vi "StateMachine_StageAutomation.vi"() -> ()   [LabVIEW 2021]
uses:
  ProgramData/PI/LabVIEW/Low Level/Communication.llb/Interface Settings.ctl
  C:/Users/csaerome/Documents/PipeJet/PipeJet/Software/bfx_piezo_r13.dll
  Documents/PipeJet/PipeJet/Software/bfx_piezo_r13.dll
panel:
  in  "Automatic2ndRow":bool
  in  "2ndRow":bool
  in  "?":bool
  out "Home Position (mm)":dbl[](array[numeric]) format="%.6f"
  in  "Home":bool
  out "Print Preview":picture
  in  "PrintPreview":bool
  in  "Num. of columns":dbl
  in  "Dist. b/w Columns (mm)":dbl[](array[numeric])
  in  "Num. of wells":dbl
  in  "Dist. b/w wells (mm)":dbl[](array[numeric])
  in  "Dist. b/w cells line (mm)":dbl[](array[numeric])
  in  "Pitch (mm)":dbl[](array[numeric])
  in  "Num. of Drops":dbl
  in  "Z-":bool
  in  "Z+":bool
  in  "Z-Step Size (mm)":dbl[](array[numeric])=[0.0]
  in  "PJ Stroke (%)":dbl
  in  "PJ Str. Velocity":dbl
  in  "SingleHead":bool
  in  "AbsCenter":bool
  in  "Position values (mm)":dbl[](array[numeric]) format="%.6f"
  in  "Y-":bool
  in  "Y+":bool
  in  "X-":bool
  in  "X+":bool
  in  "Y-Step Size (mm)":dbl[](array[numeric])=[0.0]
  out "Error Description":string
  out "error out":errorcluster
  in  "error in (no error)":errorcluster
  in  "X-Step Size (mm)":dbl[](array[numeric])=[0.0]
  out "Conn. \nAxes":string[](array[string])
  in  "Interface settings":T1={"Interface"=0, "Timeout"=5000, "RS232 settings"={"Portnumber"=6, "Baudrate"=5}, "TCP/IP settings"={"Host address/name"="localhost", "Port"=50000, "Board"=0, "TCP/IP Search?"=TRUE}, "USB settings"={"S/N"="", "USB Search?"=TRUE}, "DaisyChain settings"={"Register DC"=FALSE, "DaisyChain Search?"=TRUE, "Device ID"=1}, "DLL for Device"=0} {"DLL for Device" items=["None", "C-843", "C-844", "E-710", "C-843.PM", "C-865", "E-761", "Mercury", "E-755", "E-753", "C-866", "E-712", "E-725", "E-861", "C-867", "E-517", "E-816", "E-709", "PI_GCS2_DLL", "HydraPollux"]; "Interface" items=["RS232", "RS232 DaisyChain", "USB", "USB DaisyChain", "TCP/IP", "TCP/IP DaisyChain", "PCI"]; "RS232 settings"."Portnumber" min=1 step=1; "RS232 settings"."Baudrate" items=["9600", "14400", "19200", "38400", "57600", "115200", "230400", "460800"]}
  # "Initialization"
  # "Setup"
  # "Relative Centering"
  # "Absolute Centering"
  # "Home Settings"
  # "X:"
  # "Y:"
  # "Z:"
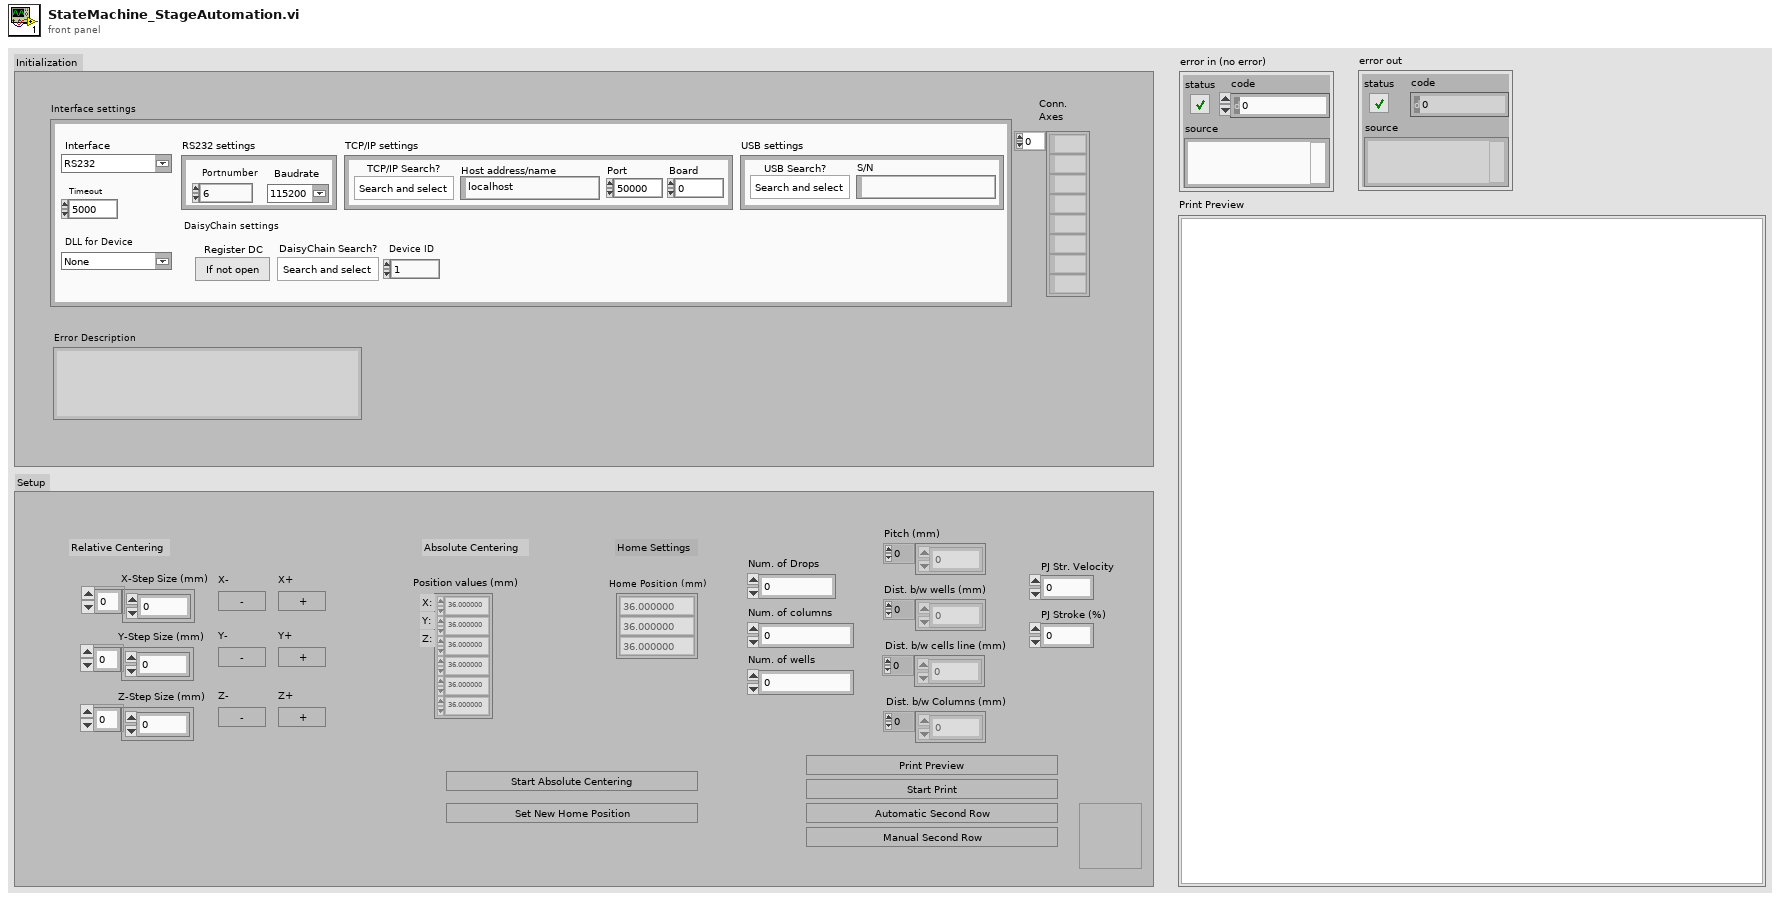
[diagram p1: front panel]
types:
  T1 = typedef "Interface Settings.ctl" = cluster{"Interface":u16, "Timeout":u32, "RS232 settings":cluster{"Portnumber":u8, "Baudrate":u16}, "TCP/IP settings":cluster{"Host address/name":string, "Port":i32, "Board":i32, "TCP/IP Search?":bool}, "USB settings":cluster{"S/N":string, "USB Search?":bool}, "DaisyChain settings":cluster{"Register DC":bool, "DaisyChain Search?":bool, "Device ID":i32}, "DLL for Device":u16}
  T2 = cluster{"Width":u16, "Style":enum32{"Solid", "Dash", "Dot", "DashDot", "DashDotDot"}}
  T3 = enum16{"Do not reference", "Reference switch", "Negative limit switch", "Positive limit switch"}[]
  T4 = cluster{"Dist. b/w cells line (mm)":dbl[], "Pitch (mm)":dbl[], "Num. of Drops":dbl, "Dist. b/w wells (mm)":dbl[], "Num. of wells":dbl, "Num. of columns":dbl, "Dist. b/w Columns (mm)":dbl[]}
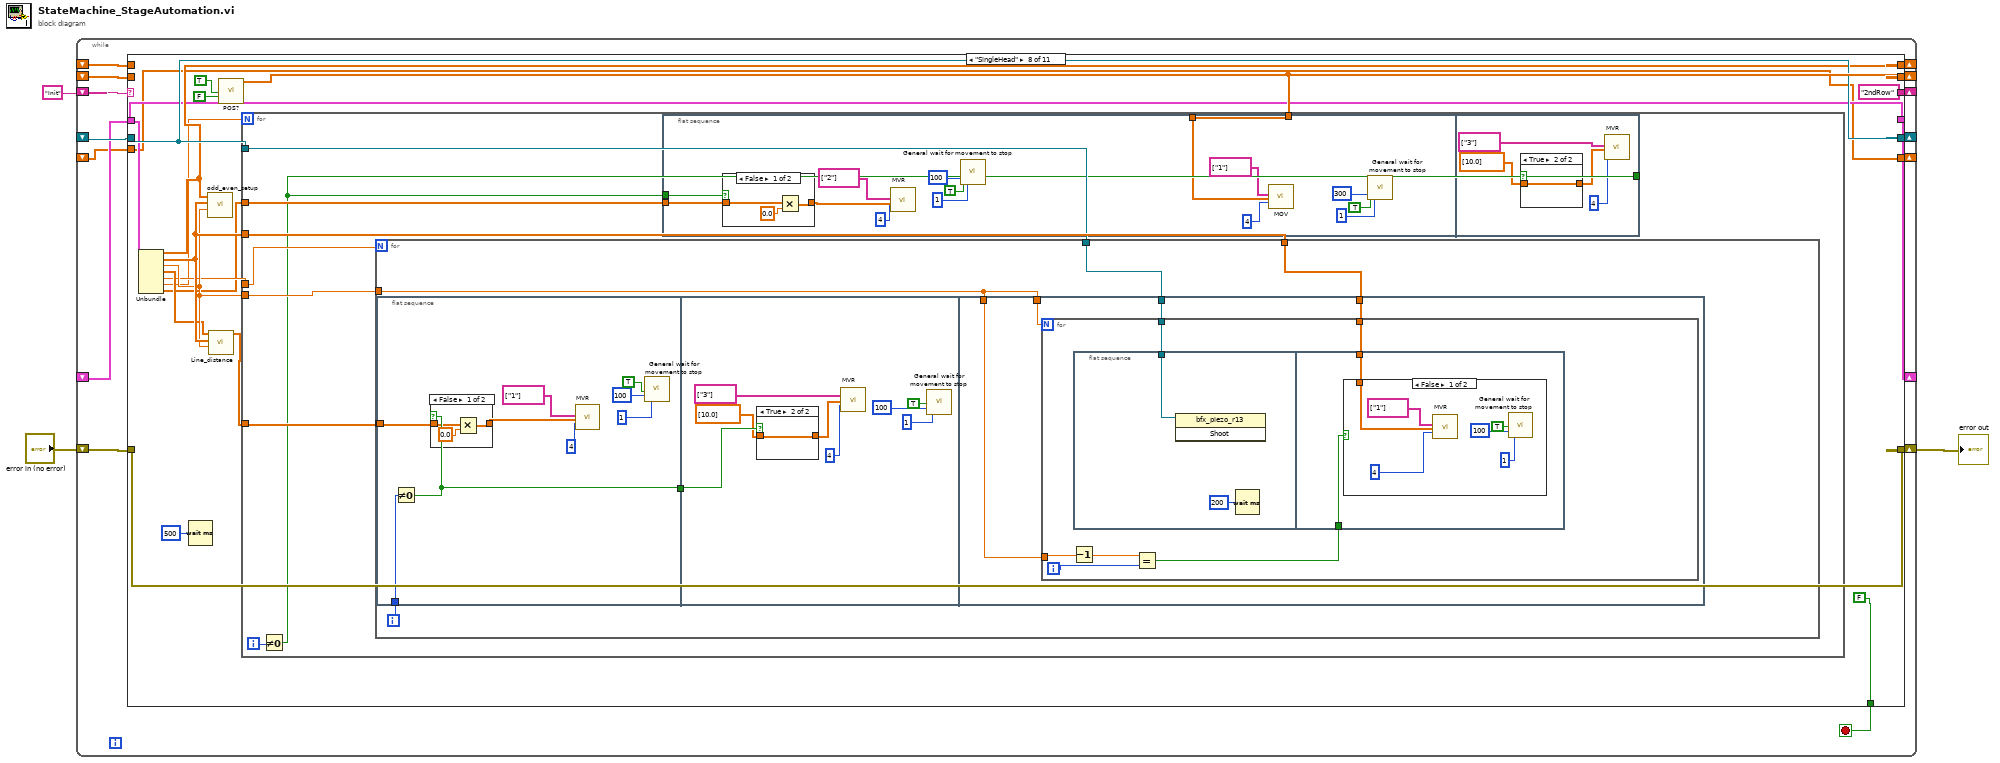
[diagram p0: block diagram]
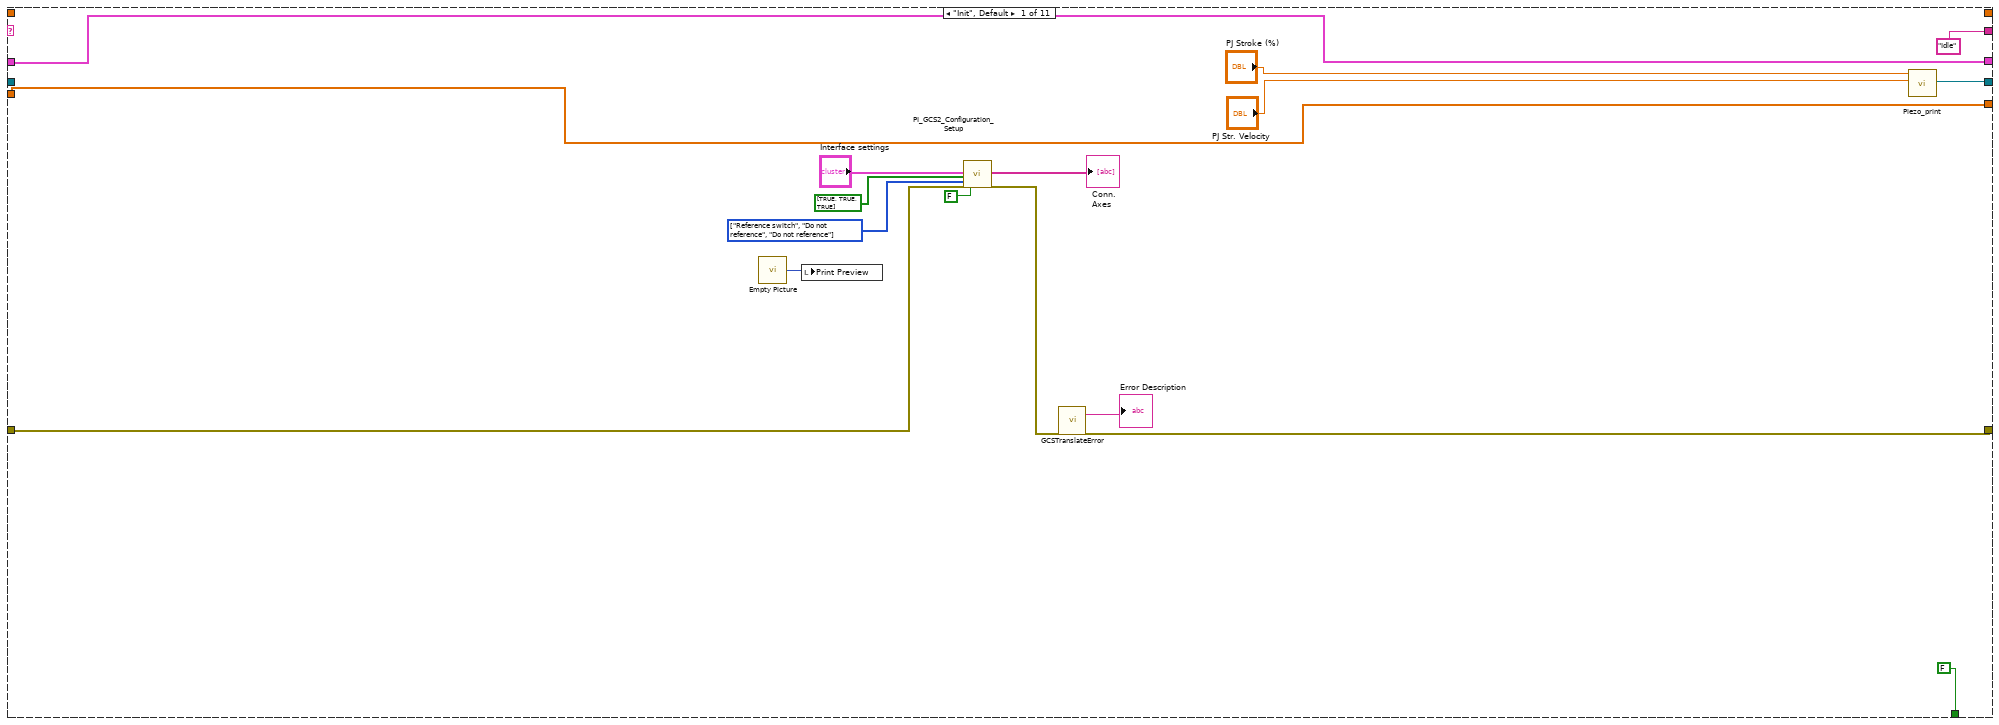
[diagram p2: hidden frame]
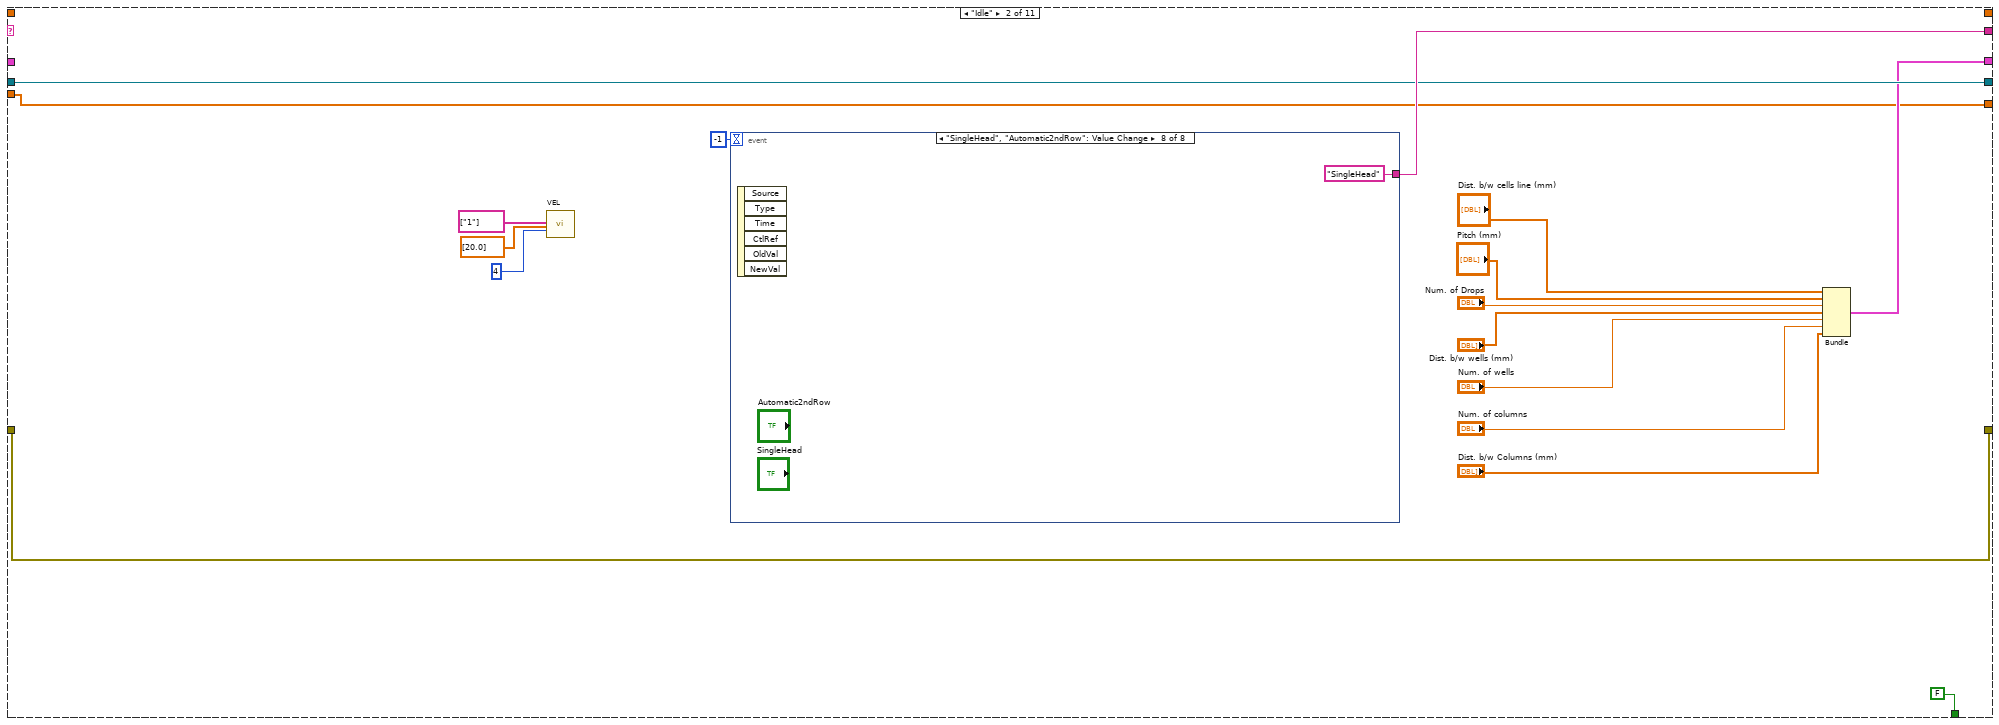
[diagram p3: hidden frame]
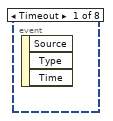
[diagram p4: hidden frame]
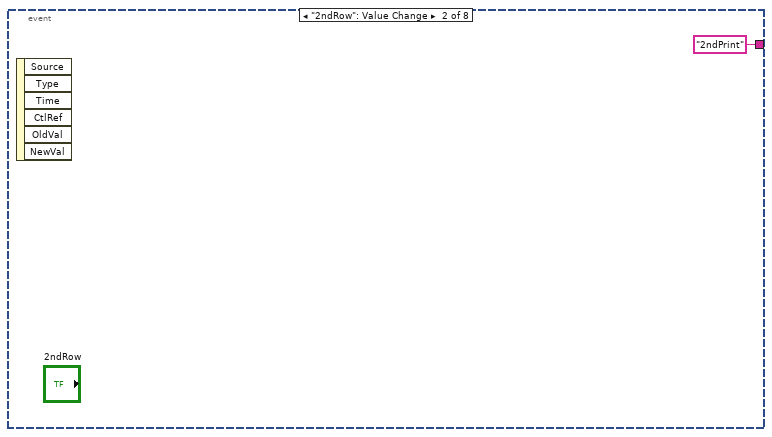
[diagram p5: hidden frame]
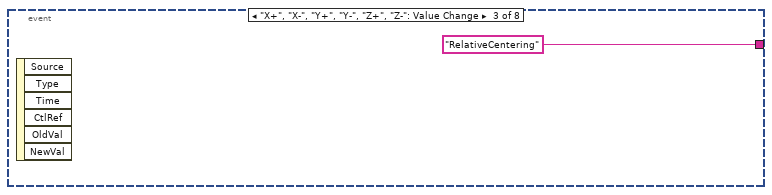
[diagram p6: hidden frame]
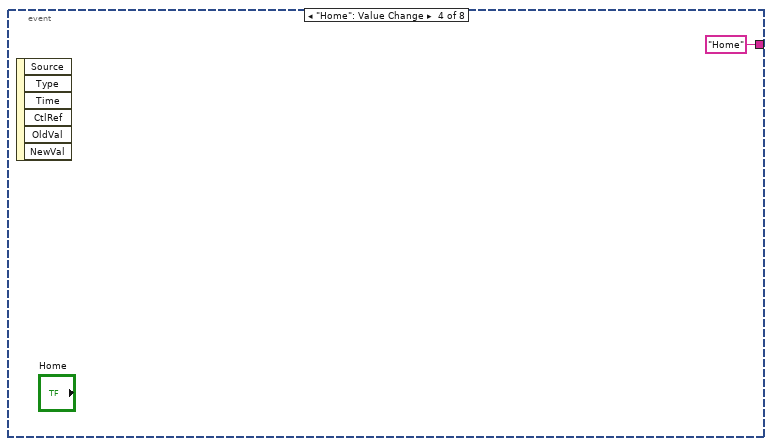
[diagram p7: hidden frame]
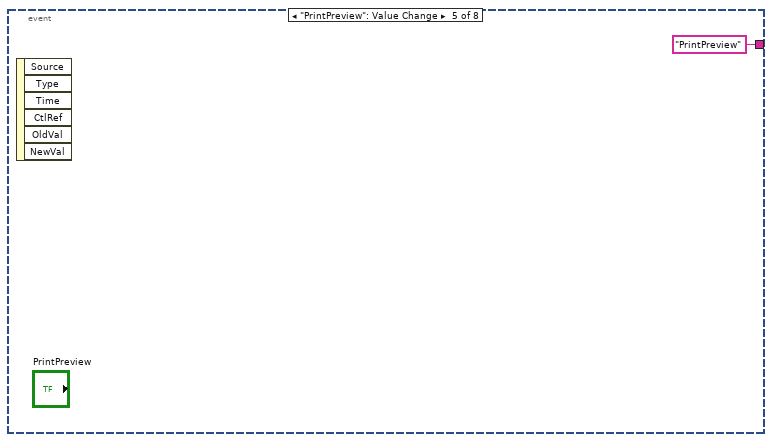
[diagram p8: hidden frame]
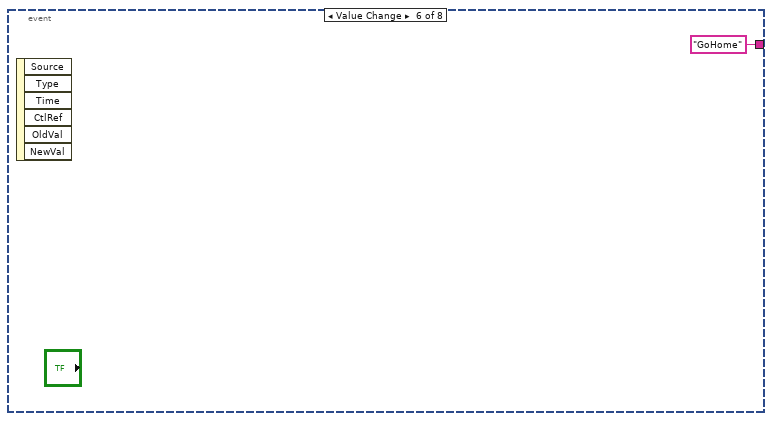
[diagram p9: hidden frame]
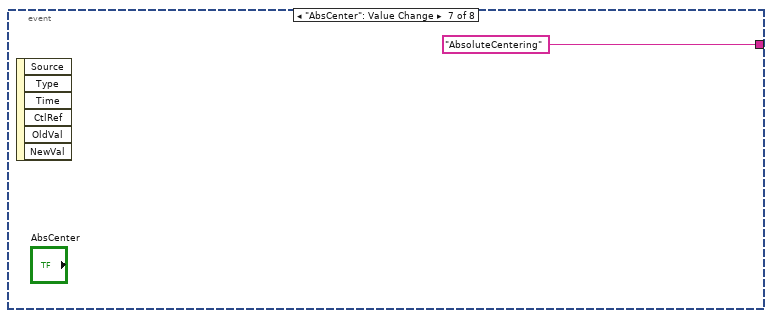
[diagram p10: hidden frame]
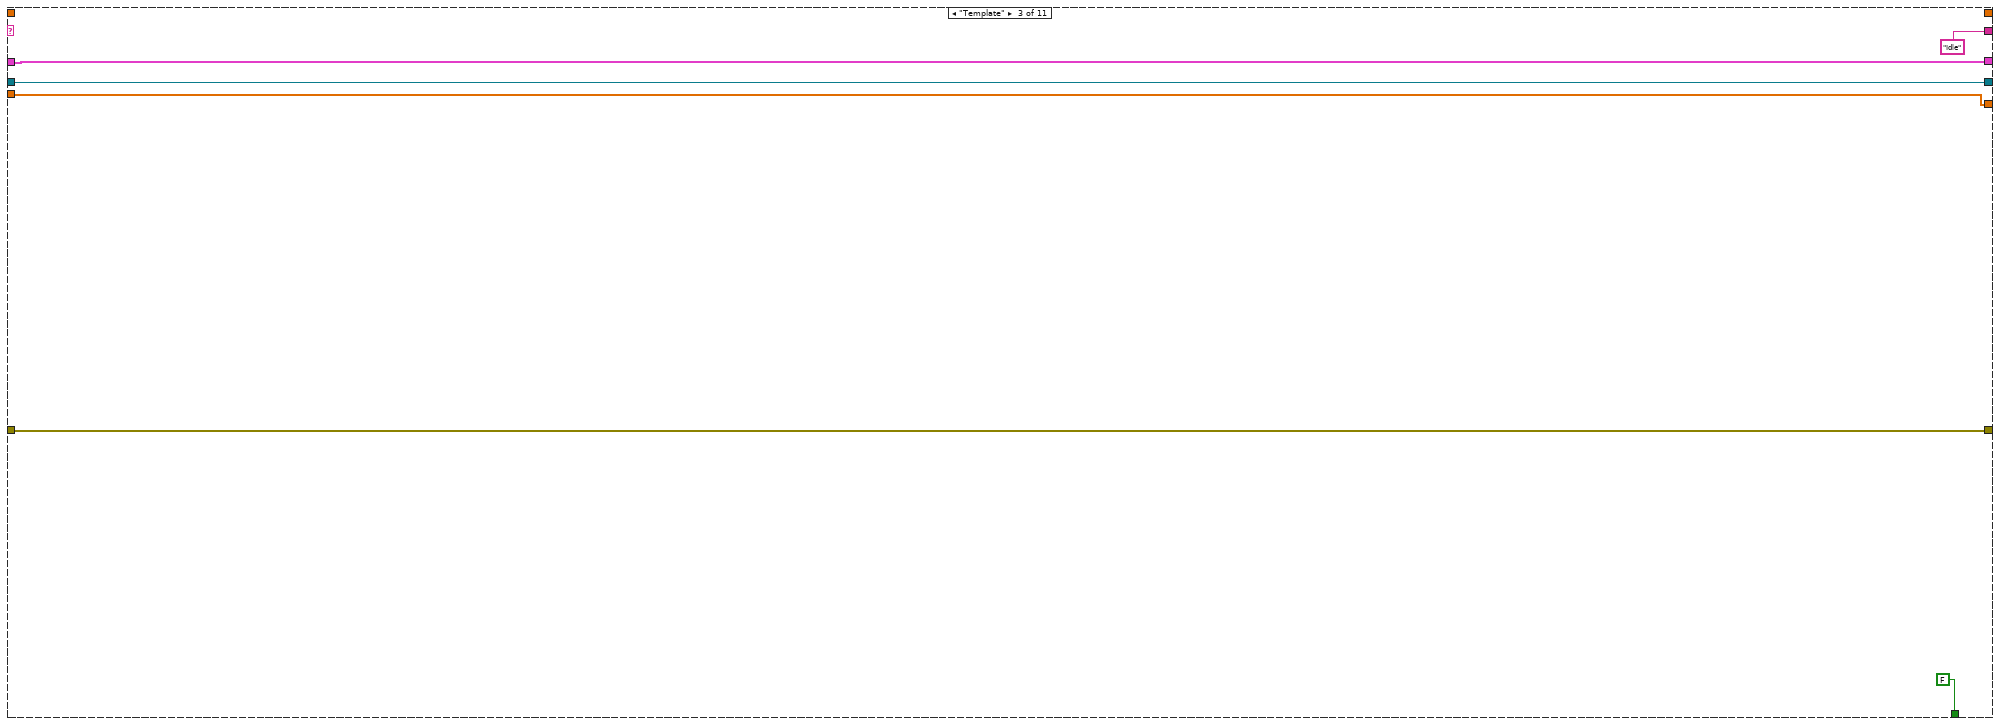
[diagram p11: hidden frame]
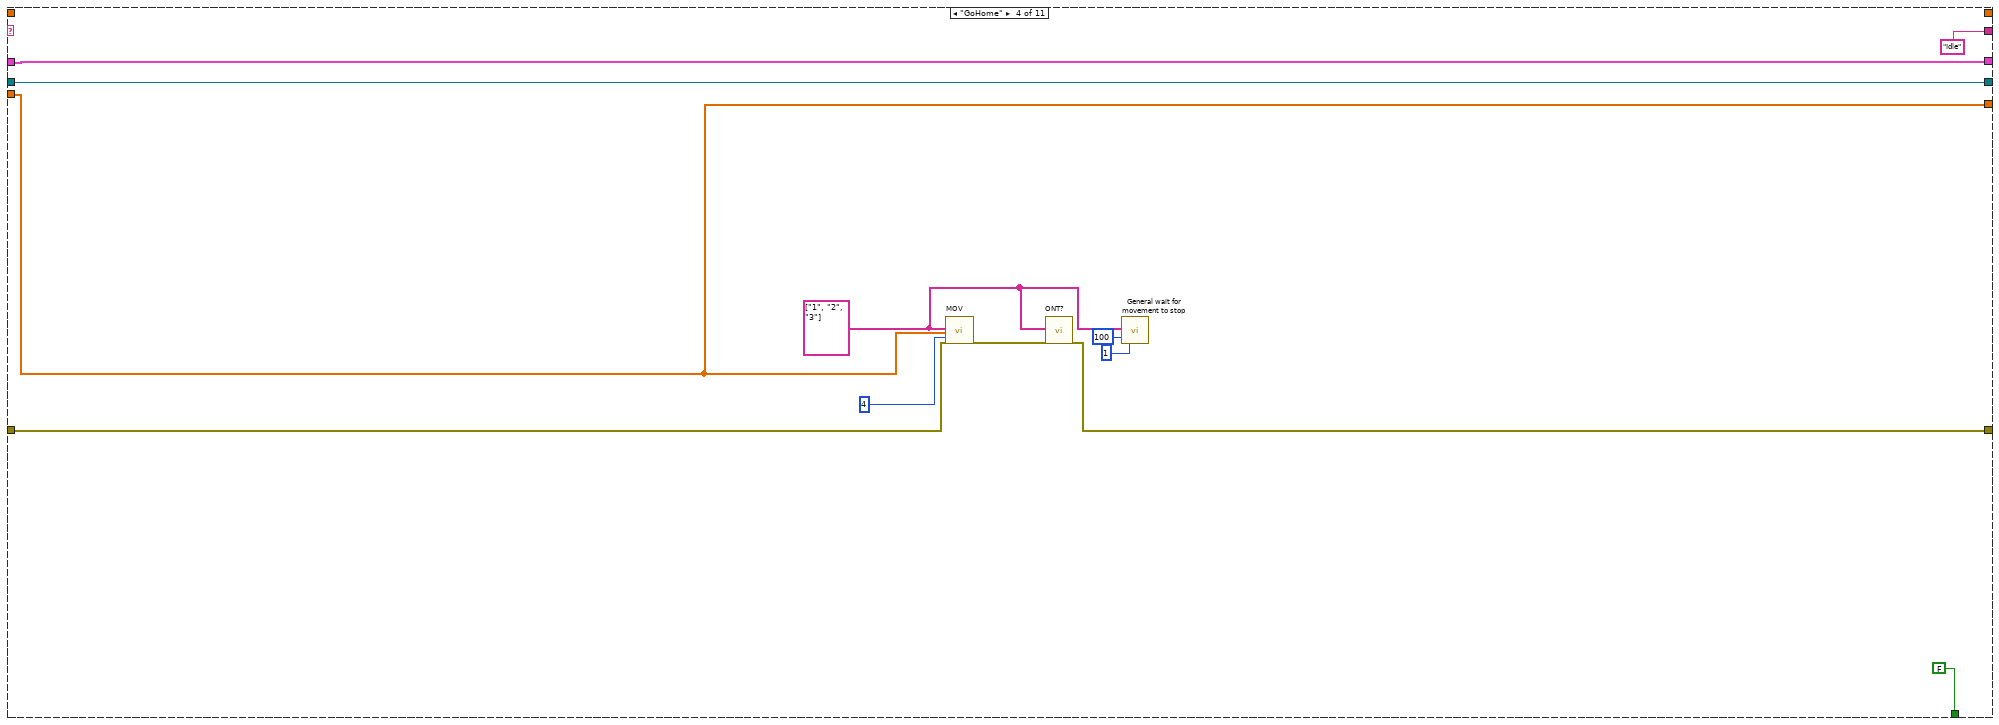
[diagram p12: hidden frame]
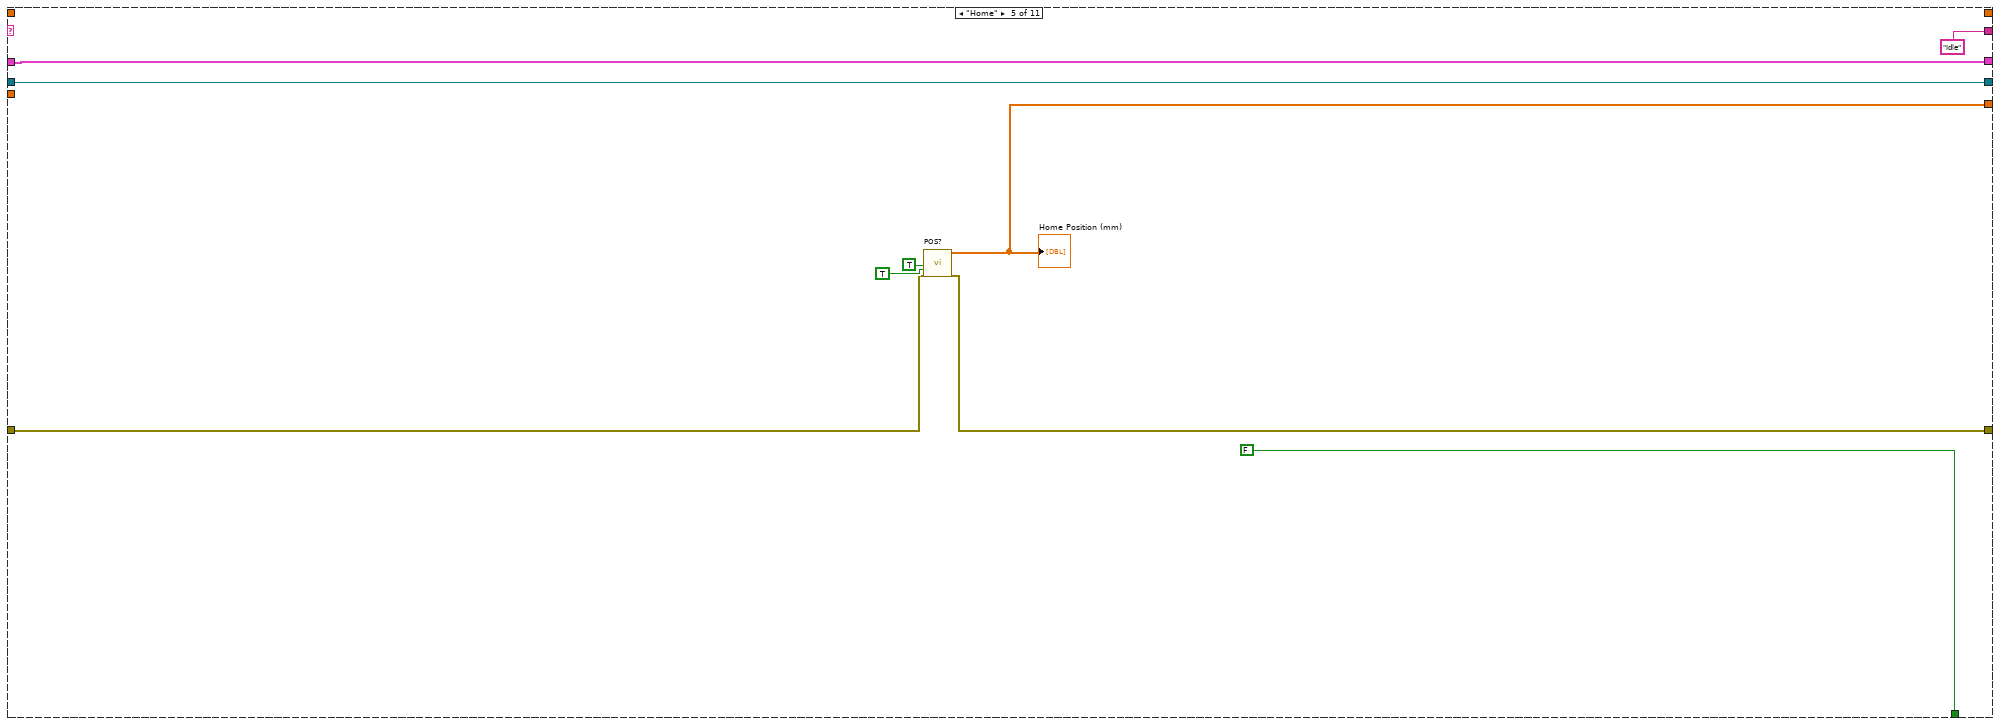
[diagram p13: hidden frame]
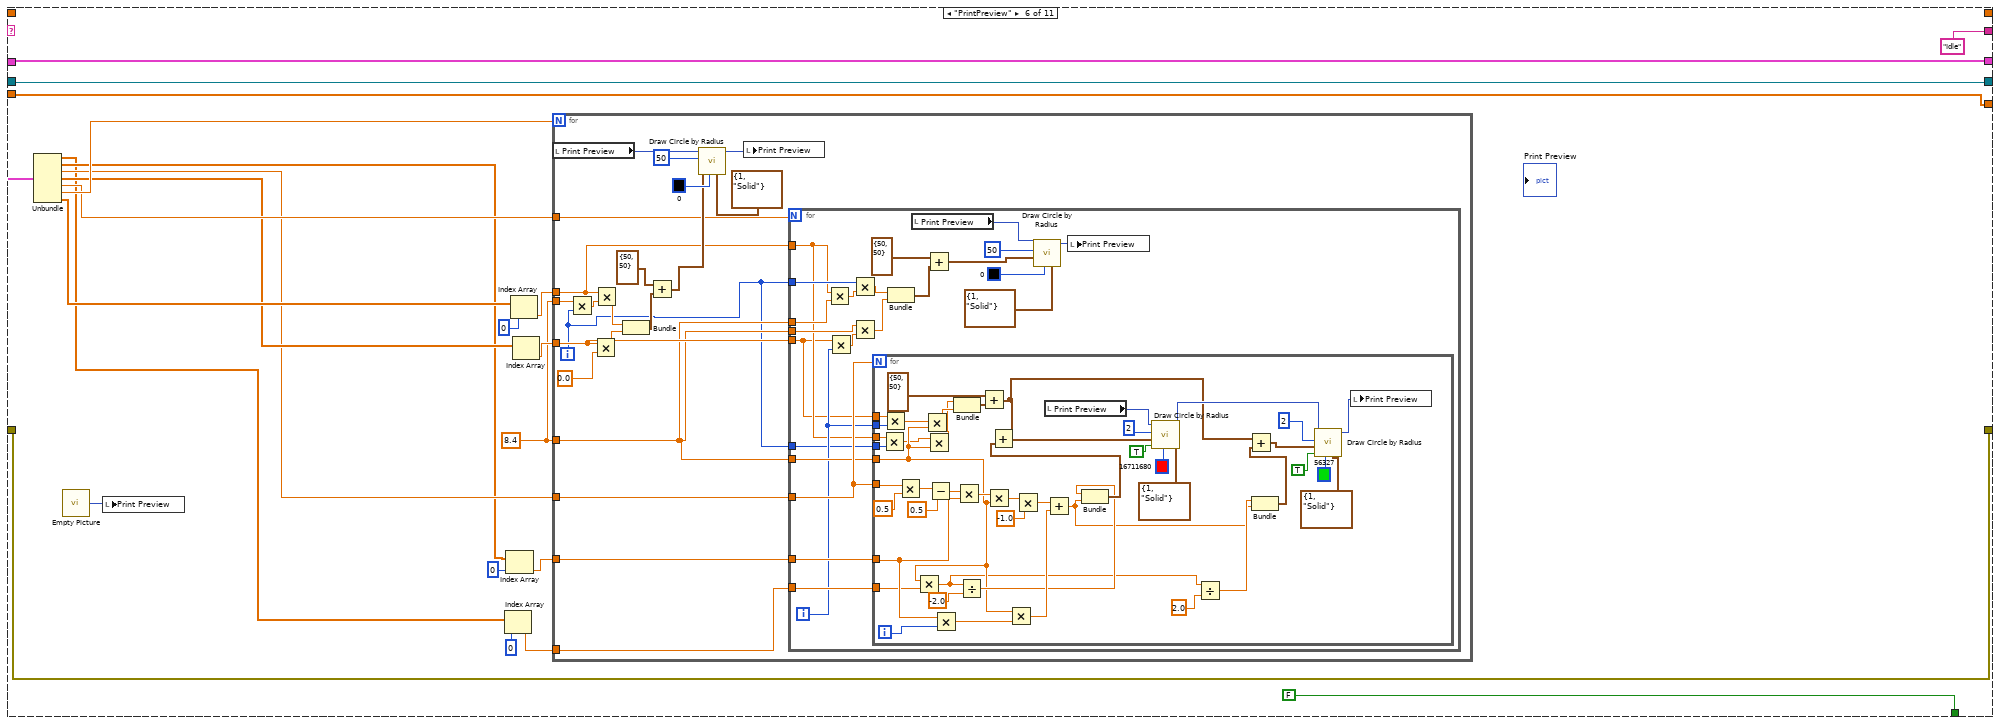
[diagram p14: hidden frame]
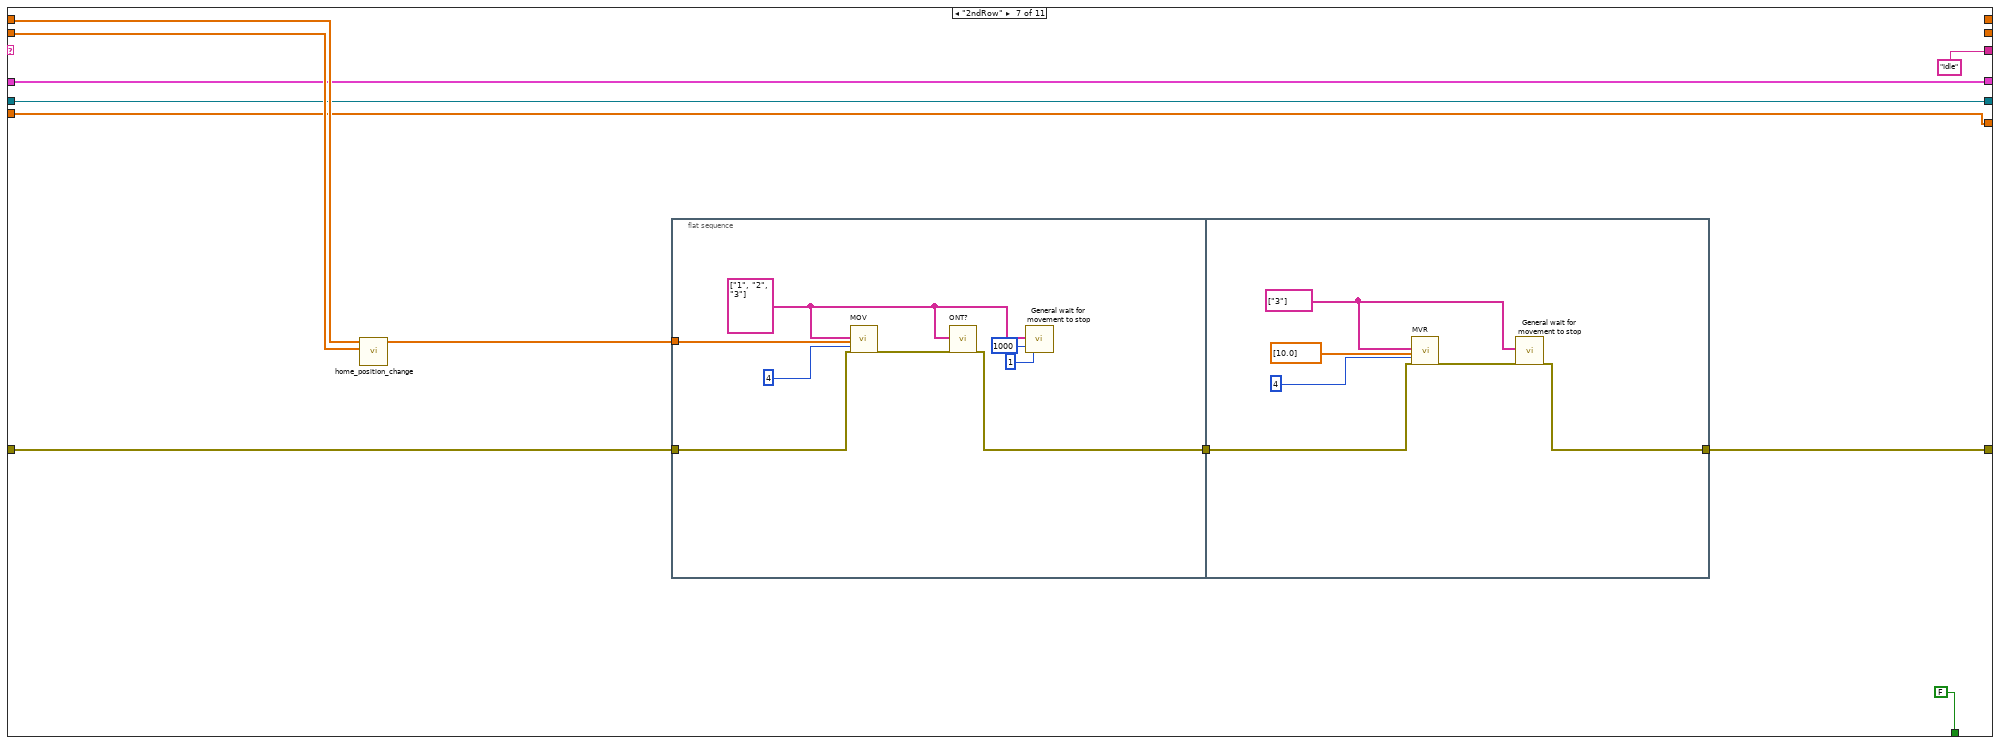
[diagram p15: hidden frame]
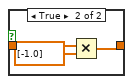
[diagram p16: hidden frame]
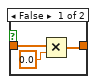
[diagram p17: hidden frame]
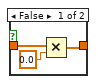
[diagram p19: hidden frame]
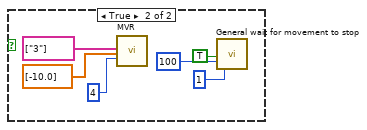
[diagram p20: hidden frame]
diagram:
  n1 = while {
    shift-right: [w17] -> w2
    shift-left: "error in (no error)" -> [w18]
    shift-right: [w15] -> _
    shift-left: "Init" -> [w16]
    shift-right: [w14] -> _
    shift-left: _ -> [w13]
    shift-right: [w12] -> _
    shift-left: _ -> [w11]
    shift-right: [w9] -> _
    shift-left: _ -> [w8]
    shift-right: [w7] -> _
    shift-left: _ -> [w6]
    shift-right: [w5] -> _
    shift-left: _ -> [w4]
    stop <- w10 stop-if-true
    n2 = case shown="\"SingleHead\"" w16 {
      tunnel: [FALSE FALSE FALSE FALSE FALSE FALSE FALSE FALSE FALSE FALSE FALSE] -> w10
      tunnel: w18 -> [w30 w51 w64 w68 w80 w107 w208 w241 w354 w446 w480]
      tunnel: [w29 w51 w64 w67 w79 w107 w207 w241 w354 w445 w480] -> w17
      tunnel: ["Idle" w49 "Idle" "Idle" "Idle" "Idle" "Idle" "2ndRow" "2ndRow" "Idle" "Idle"] -> w15
      tunnel: [_ _ _ _ _ _ _ w237 w350 _ _] -> w14
      tunnel: w13 -> [_ _ _ _ _ _ w206 _ _ _ _]
      tunnel: [_ _ _ _ _ _ _ w233 w346 _ _] -> w12
      tunnel: w11 -> [_ _ _ _ _ _ w204 _ _ _ _]
      tunnel: [w23 w48 w62 w75 w84 w105 w203 w234 w347 w442 w478] -> w9
      tunnel: w8 -> [_ w48 w62 w75 w84 w105 w203 w234 w347 w442 w478]
      tunnel: [w22 w45 w61 w74 w83 w104 w202 w226 w339 w441 w477] -> w7
      tunnel: w6 -> [w22 _ w61 w74 w83 w104 w202 w226 w339 w441 w477]
      tunnel: [w20 w39 w60 w66 w78 w87 w201 w225 w338 w439 w476] -> w5
      tunnel: w4 -> [w20 w39 w60 w66 _ w87 w201 w225 w338 w439 w476]
      frame "Init", Default {
        w32 = T3 [enum."Reference switch", enum."Do not reference", enum."Do not reference"] items=["Do not reference", "Reference switch", "Negative limit switch", "Positive limit switch"] ("Reference mode")
        n3 = call "Empty Picture"() -> ("empty picture"=w21:picture)
        n4 = local write "Print Preview"(w21) -> ()
        n5 = call "PI_GCS2_Configuration_Setup.vi"("Interface settings"="Interface settings", "Closed Loop"=bool[] [TRUE, TRUE, TRUE], "Reference mode"=w32, "error in"=w30, "Stop all motion?\n(#24)"=FALSE ("Stop all motion?\n(#24)")) -> ("Conn. \nAxes"=→"Conn. \nAxes":string[], "error out"=w27:errorcluster)  [unwired: 3 in, 10 out]
        n6 = call "GCSTranslateError.vi"("error in"=w27) -> ("Error Description"=→"Error Description":string, "error out"=w29:errorcluster)  [unwired: 17 out]
        n7 = call "Piezo_print.vi"("DownStrokeVelocity"="PJ Str. Velocity", "StrokeLength"="PJ Stroke (%)") -> (".NET Refnum out"=w23:refnum<k24>)  [unwired: 9 in]
      }
      frame "Idle" {
        n8 = call "VEL.vi"("Axes to set"=string[] ["1"], "Velocity values"=dbl[] [20.0], "No.of digits"=i16 4) -> ()  [unwired: 3 in, 14 out]
        n9 = event shown="[7] \"SingleHead\", \"Automatic2ndRow\": Value Change" {
          selector: _ -> [_ _ _ _ _ _ _ _]
          dyn-events: _ -> [_ _ _ _ _ _ _ _]
          timeout: -1 -> [_ _ _ _ _ _ _ _]
          tunnel: [_ "2ndPrint" "RelativeCentering" "Home" "PrintPreview" "GoHome" "AbsoluteCentering" "SingleHead"] -> w49
          event Timeout {
            n10 = event-data() -> ()  [unwired: 1 in, 3 out]
          }
          event "2ndRow": Value Change {
            n11 = event-data() -> ()  [unwired: 1 in, 6 out]
          }
          event "X+", "X-", "Y+", "Y-", "Z+", "Z-": Value Change {
            n12 = event-data() -> ()  [unwired: 1 in, 6 out]
          }
          event "Home": Value Change {
            n13 = event-data() -> ()  [unwired: 1 in, 6 out]
          }
          event "PrintPreview": Value Change {
            n14 = event-data() -> ()  [unwired: 1 in, 6 out]
          }
          event Value Change {
            n15 = event-data() -> ()  [unwired: 1 in, 6 out]
          }
          event "AbsCenter": Value Change {
            n16 = event-data() -> ()  [unwired: 1 in, 6 out]
          }
          event "SingleHead", "Automatic2ndRow": Value Change {
            n17 = event-data() -> ()  [unwired: 1 in, 6 out]
          }
        }
        n18 = Bundle("Dist. b/w cells line (mm)"="Dist. b/w cells line (mm)", "Pitch (mm)"="Pitch (mm)", "Num. of Drops"="Num. of Drops", "Dist. b/w wells (mm)"="Dist. b/w wells (mm)", "Num. of wells"="Num. of wells", "Num. of columns"="Num. of columns", "Dist. b/w Columns (mm)"="Dist. b/w Columns (mm)") -> (w45:T4)  [unwired: 1 in]
      }
      frame "Template" {
      }
      frame "GoHome" {
        w69 = string[] ["1", "2", "3"] ("Axes to move")
        n19 = call "MOV.vi"("Axes to move"=w69, "Position values"=w66, "No.of digits"=i16 4, "error in"=w68) -> ("error out"=w73:errorcluster)  [unwired: 1 in, 14 out]
        n20 = call "ONT?.vi"("Axes to query"=w69, "error in"=w73) -> ("error out"=w67:errorcluster)  [unwired: 3 in, 14 out]
        n21 = call "General wait for movement to stop.vi"("Axes to wait for"=w69, "Additional wait time, ms"=u32 100, "Polling cycle \ntime, ms"=u32 1 ("Polling cycle \ntime, ms")) -> ()  [unwired: 5 in, 12 out]
      }
      frame "Home" {
        n22 = call "POS?.vi"("All axes?"=TRUE, "Axis identifier?"=TRUE, "error in"=w80) -> ("Position"=w78:dbl[], "error out"=w79:errorcluster)  [unwired: 2 in, 13 out]
        "Home Position (mm)" <- w78
      }
      frame "PrintPreview" {
        w89 = 8.4 ("Scale")
        n23 = Unbundle(w104) -> ("Dist. b/w cells line (mm)"=w90:dbl[], "Pitch (mm)"=w91:dbl[], "Num. of Drops"=w92:dbl, "Dist. b/w wells (mm)"=w93:dbl[], "Num. of wells"=w95:dbl, "Num. of columns"=w96:dbl, "Dist. b/w Columns (mm)"=w94:dbl[])
        n24 = call "Empty Picture"() -> ("empty picture"=w88:picture)
        n25 = local write "Print Preview"(w88) -> ()
        n26 = Index Array(array=w90, index=0) -> (element=w97:dbl)
        n27 = Index Array(array=w91, index=0) -> (element=w100:dbl)
        n28 = Index Array(array=w94, index=0) -> (element=w102:dbl)
        n29 = Index Array(array=w93) -> (element=w101:dbl)  [unwired: 1 in]
        n30 = for {
          N: w96 -> [_]
          tunnel: w101 -> [w118]
          tunnel: w102 -> [w115]
          tunnel: w95 -> [w119]
          tunnel: w89 -> [w114]
          tunnel: w89 -> [w110]
          tunnel: w92 -> [w113]
          tunnel: w100 -> [w112]
          tunnel: w97 -> [w111]
          i -> [w109]
          n31 = local read "Print Preview"() -> (w123:picture)
          n32 = Multiply(x=w114, y=w109) -> (x*y=w120:dbl)
          n33 = Multiply(x=w118, y=0.0) -> (x*y=w122:dbl)
          n34 = Multiply(x=w115, y=w120) -> (x*y=w117:dbl)
          n35 = Bundle(w117, w122) -> (w124:cluster{dbl, dbl})  [unwired: 1 in]
          n36 = Add(x=cluster{"horizontal":i16, "vertical":i16} {"horizontal"=50, "vertical"=50} ("pixel center"), y=w124) -> (x+y=w125:cluster{dbl, dbl})
          n37 = call <vilib>:"Draw Circle by Radius.vi"("pen"=T2 {"Width"=1, "Style"=enum."Solid"}, "color(black)"=u32 0, "pixel center"=w125, "radius"=i16 50, "picture"=w123) -> ("new picture"=w116:picture)  [unwired: 6 in]
          n38 = local write "Print Preview"(w116) -> ()
          n39 = for {
            N: w119 -> [_]
            tunnel: w118 -> [w130]
            tunnel: w115 -> [w131]
            tunnel: w109 -> [w140]
            tunnel: w110 -> [w139]
            tunnel: w110 -> [w138]
            tunnel: w113 -> [w137]
            tunnel: w112 -> [w136]
            tunnel: w111 -> [w135]
            tunnel: w110 -> [w134]
            tunnel: w109 -> [w132]
            i -> [w133]
            n40 = Multiply(x=w131, y=w139) -> (x*y=w141:dbl)
            n41 = Multiply(x=w130, y=w133) -> (x*y=w144:dbl)
            n42 = Multiply(x=w140, y=w141) -> (x*y=w145:dbl)
            n43 = Multiply(x=w138, y=w144) -> (x*y=w146:dbl)
            n44 = for {
              N: w137 -> [_]
              tunnel: w137 -> [w188]
              tunnel: w136 -> [w180]
              tunnel: w135 -> [w173]
              tunnel: w134 -> [w168]
              tunnel: w133 -> [w165]
              tunnel: w132 -> [w164]
              tunnel: w131 -> [w154]
              tunnel: w130 -> [w153]
              i -> [w181]
              n45 = Multiply(x=w154, y=w164) -> (x*y=w166:dbl)
              n46 = Multiply(x=w153, y=w165) -> (x*y=w167:dbl)
              n47 = Multiply(x=w188, y=0.5) -> (x*y=w187:dbl)
              n48 = Multiply(x=w168, y=w173) -> (x*y=w157:dbl)
              n49 = Multiply(x=w167, y=w168) -> (x*y=w163:dbl)
              n50 = Multiply(x=w166, y=w168) -> (x*y=w162:dbl)
              n51 = Subtract(x=w187, y=0.5) -> (x-y=w184:dbl)
              n52 = Multiply(x=w180, y=w181) -> (x*y=w175:dbl)
              n53 = Bundle(w162, w163) -> (w170:cluster{dbl, dbl})  [unwired: 1 in]
              n54 = Multiply(x=w184, y=w180) -> (x*y=w183:dbl)
              n55 = Divide(x=w157, y=-2.0) -> (x/y=w171:dbl)
              n56 = Add(x=cluster{"horizontal":i16, "vertical":i16} {"horizontal"=50, "vertical"=50} ("pixel center"), y=w170) -> (x+y=w160:cluster{dbl, dbl})
              n57 = Multiply(x=w183, y=w168) -> (x*y=w179:dbl)
              n58 = Multiply(x=w168, y=w175) -> (x*y=w174:dbl)
              n59 = Multiply(x=w179, y=-1.0) -> (x*y=w177:dbl)
              n60 = local read "Print Preview"() -> (w198:picture)
              n61 = Add(x=w177, y=w174) -> (x+y=w155:dbl)
              n62 = Bundle(w171, w155) -> (w182:cluster{dbl, dbl})  [unwired: 1 in]
              n63 = Add(x=w160, y=w182) -> (x+y=w176:cluster{dbl, dbl})
              n64 = call <vilib>:"Draw Circle by Radius.vi"("pen"=T2 {"Width"=1, "Style"=enum."Solid"}, "color(black)"=u32 16711680, "fill?(F)"=TRUE, "pixel center"=w176, "radius"=i16 2, "picture"=w198) -> ("new picture"=w190:picture)  [unwired: 5 in]
              n65 = Divide(x=w157, y=2.0) -> (x/y=w156:dbl)
              n66 = Bundle(w156, w155) -> (w159:cluster{dbl, dbl})  [unwired: 1 in]
              n67 = Add(x=w160, y=w159) -> (x+y=w161:cluster{dbl, dbl})
              n68 = call <vilib>:"Draw Circle by Radius.vi"("pen"=T2 {"Width"=1, "Style"=enum."Solid"}, "color(black)"=u32 56327, "fill?(F)"=TRUE, "pixel center"=w161, "radius"=i16 2, "picture"=w190) -> ("new picture"=w189:picture)  [unwired: 5 in]
              n69 = local write "Print Preview"(w189) -> ()
            }
            n70 = Bundle(w145, w146) -> (w147:cluster{dbl, dbl})  [unwired: 1 in]
            n71 = local read "Print Preview"() -> (w142:picture)
            n72 = Add(x=cluster{"horizontal":i16, "vertical":i16} {"horizontal"=50, "vertical"=50} ("pixel center"), y=w147) -> (x+y=w149:cluster{dbl, dbl})
            n73 = call <vilib>:"Draw Circle by Radius.vi"("pen"=T2 {"Width"=1, "Style"=enum."Solid"}, "color(black)"=u32 0, "pixel center"=w149, "radius"=i16 50, "picture"=w142) -> ("new picture"=w143:picture)  [unwired: 6 in]
            n74 = local write "Print Preview"(w143) -> ()
          }
        }
      }
      frame "2ndRow" {
        n75 = call "home_position_change.vi"("Position"=w206, "Dist. b/w cells line"=w204) -> ("Array"=w205:dbl[])  [unwired: 9 in]
        n76 = flat-sequence {
          tunnel: w208 -> [w216]
          tunnel: w205 -> [w212]
          tunnel: [w215] -> w200
          tunnel: [w219] -> w207
          tunnel: w200 -> [w224]
          frame #0 {
            w214 = string[] ["1", "2", "3"] ("Axes to move")
            n77 = call "MOV.vi"("Axes to move"=w214, "Position values"=w212, "No.of digits"=i16 4, "error in"=w216) -> ("error out"=w218:errorcluster)  [unwired: 1 in, 14 out]
            n78 = call "ONT?.vi"("Axes to query"=w214, "error in"=w218) -> ("error out"=w215:errorcluster)  [unwired: 3 in, 14 out]
            n79 = call "General wait for movement to stop.vi"("Axes to wait for"=w214, "Additional wait time, ms"=u32 1000, "Polling cycle \ntime, ms"=u32 1 ("Polling cycle \ntime, ms")) -> ()  [unwired: 5 in, 12 out]
          }
          frame #1 {
            w221 = string[] ["3"] ("Axes to move")
            n80 = call "MVR.vi"("Axes to move"=w221, "Position values"=dbl[] [10.0], "No.of digits"=i16 4, "error in"=w224) -> ("error out"=w220:errorcluster)  [unwired: 1 in, 14 out]
            n81 = call "General wait for movement to stop.vi"("Axes to wait for"=w221, "error in"=w220) -> ("error out"=w219:errorcluster)  [unwired: 6 in, 11 out]
          }
        }
      }
      frame "SingleHead" {
        n82 = Unbundle(w226) -> ("Dist. b/w cells line (mm)"=w233:dbl[], "Pitch (mm)"=w232:dbl[], "Num. of Drops"=w231:dbl, "Dist. b/w wells (mm)"=w230:dbl[], "Num. of wells"=w229:dbl, "Num. of columns"=w228:dbl, "Dist. b/w Columns (mm)"=w227:dbl[])
        n83 = Wait (ms)(milliseconds to wait=u32 500) -> ()  [unwired: 1 out]
        n84 = call "odd_even_setup.vi"("Num. of Drops in"=w231, "Pitch in"=w232, "Distance b/w cells in"=w233) -> ()  [unwired: 9 in]
        n85 = call "Line_distance.vi"("Num. of Drops in"=w231, "Pitch in"=w232, "Dist. b/w Lines in"=w230) -> ("Array"=w236:dbl[])  [unwired: 8 in]
        n86 = call "POS?.vi"("All axes?"=TRUE, "Axis identifier?"=FALSE) -> ("Position"=w237:dbl[])  [unwired: 3 in, 14 out]
        n87 = for {
          N: w228 -> [_]
          tunnel: w237 -> [w247]
          tunnel: w231 -> [w250]
          tunnel: w232 -> [w249]
          tunnel: w236 -> [w248]
          tunnel: w234 -> [w246]
          tunnel: w229 -> [w245]
          tunnel: w227 -> [w244]
          i -> [w251]
          n88 = Not Equal To 0?(x=w251) -> (x != 0?=w243:bool)
          n89 = for {
            N: w245 -> [_]
            tunnel: w250 -> [w281]
            tunnel: w249 -> [w285]
            tunnel: w248 -> [w284]
            tunnel: w246 -> [w283]
            i -> [w286]
            n90 = flat-sequence {
              tunnel: w286 -> [w289]
              tunnel: w284 -> [w288]
              tunnel: [w287] -> w282
              tunnel: w282 -> [w302]
              tunnel: w281 -> [w315]
              tunnel: w285 -> [w314]
              tunnel: w283 -> [w313]
              tunnel: w281 -> [w312]
              frame #0 {
                n91 = Not Equal To 0?(x=w289) -> (x != 0?=w287:bool)
                n92 = case shown="False" w287 {
                  tunnel: w288 -> [w297 w299]
                  tunnel: [w296 w299] -> w291
                  frame False {
                    n93 = Multiply(x=w297, y=0.0) -> (x*y=w296:dbl[])
                  }
                  frame True {
                  }
                }
                n94 = call "MVR.vi"("Axes to move"=string[] ["1"], "Position values"=w291, "No.of digits"=i16 4) -> ()  [unwired: 2 in, 15 out]
                n95 = call "General wait for movement to stop.vi"("All axes?"=TRUE, "Additional wait time, ms"=u32 100, "Polling cycle \ntime, ms"=u32 1 ("Polling cycle \ntime, ms")) -> ()  [unwired: 5 in, 12 out]
              }
              frame #1 {
                n96 = case shown="True" w302 {
                  tunnel: dbl[] [10.0] ("Position values") -> [w309 w311]
                  tunnel: [w308 w311] -> w300
                  frame False {
                    n97 = Multiply(x=w309, y=0.0) -> (x*y=w308:dbl[])
                  }
                  frame True {
                  }
                }
                n98 = call "MVR.vi"("Axes to move"=string[] ["3"], "Position values"=w300, "No.of digits"=i16 4) -> ()  [unwired: 2 in, 15 out]
                n99 = call "General wait for movement to stop.vi"("All axes?"=TRUE, "Additional wait time, ms"=u32 100, "Polling cycle \ntime, ms"=u32 1 ("Polling cycle \ntime, ms")) -> ()  [unwired: 5 in, 12 out]
              }
              frame #2 {
                n100 = for {
                  N: w315 -> [_]
                  tunnel: w314 -> [w319]
                  tunnel: w313 -> [w318]
                  tunnel: w312 -> [w316]
                  i -> [w321]
                  n101 = Decrement(x=w316) -> (x-1=w317:dbl)
                  n102 = flat-sequence {
                    tunnel: w318 -> [w322]
                    tunnel: w320 -> [w325]
                    tunnel: w319 -> [w324]
                    frame #0 {
                      n103 = invoke class="bfx_piezo_r13" method="Shoot"(reference=w322) -> ()  [unwired: 2 in, 3 out]
                      n104 = Wait (ms)(milliseconds to wait=u32 200) -> ()  [unwired: 1 out]
                    }
                    frame #1 {
                      n105 = case shown="False" w325 {
                        tunnel: w324 -> [w326 _]
                        frame False {
                          n106 = call "MVR.vi"("Axes to move"=string[] ["1"], "Position values"=w326, "No.of digits"=i16 4) -> ()  [unwired: 2 in, 15 out]
                          n107 = call "General wait for movement to stop.vi"("All axes?"=TRUE, "Additional wait time, ms"=u32 100, "Polling cycle \ntime, ms"=u32 1 ("Polling cycle \ntime, ms")) -> ()  [unwired: 5 in, 12 out]
                        }
                        frame True {
                          n108 = call "MVR.vi"("Axes to move"=string[] ["3"], "Position values"=dbl[] [-10.0], "No.of digits"=i16 4) -> ()  [unwired: 2 in, 15 out]
                          n109 = call "General wait for movement to stop.vi"("All axes?"=TRUE, "Additional wait time, ms"=u32 100, "Polling cycle \ntime, ms"=u32 1 ("Polling cycle \ntime, ms")) -> ()  [unwired: 5 in, 12 out]
                        }
                      }
                    }
                  }
                  n110 = Equal?(x=w317, y=w321) -> (x = y?=w320:bool)
                }
              }
            }
          }
          n111 = flat-sequence {
            tunnel: w247 -> [w254]
            tunnel: w244 -> [w253]
            tunnel: w243 -> [w252]
            tunnel: w243 -> [w275]
            frame #0 {
              n112 = case shown="False" w252 {
                tunnel: w253 -> [w267 w271]
                tunnel: [w266 w270] -> w261
                frame False {
                  n113 = Multiply(x=w267, y=0.0) -> (x*y=w266:dbl[])
                }
                frame True {
                  n114 = Multiply(x=w271, y=dbl[] [-1.0]) -> (x*y=w270:dbl[])
                }
              }
              n115 = call "MVR.vi"("Axes to move"=string[] ["2"], "Position values"=w261, "No.of digits"=i16 4) -> ()  [unwired: 2 in, 15 out]
              n116 = call "General wait for movement to stop.vi"("All axes?"=TRUE, "Additional wait time, ms"=u32 100, "Polling cycle \ntime, ms"=u32 1 ("Polling cycle \ntime, ms")) -> ()  [unwired: 5 in, 12 out]
              n117 = call "MOV.vi"("Axes to move"=string[] ["1"], "Position values"=w254, "No.of digits"=i16 4) -> ()  [unwired: 2 in, 15 out]
              n118 = call "General wait for movement to stop.vi"("All axes?"=TRUE, "Additional wait time, ms"=u32 300, "Polling cycle \ntime, ms"=u32 1 ("Polling cycle \ntime, ms")) -> ()  [unwired: 5 in, 12 out]
            }
            frame #1 {
              n119 = case shown="True" w275 {
                tunnel: dbl[] [10.0] ("Position values") -> [w278 w280]
                tunnel: [w277 w280] -> w276
                frame False {
                  n120 = Multiply(x=w278, y=0.0) -> (x*y=w277:dbl[])
                }
                frame True {
                }
              }
              n121 = call "MVR.vi"("Axes to move"=string[] ["3"], "Position values"=w276, "No.of digits"=i16 4) -> ()  [unwired: 2 in, 15 out]
            }
          }
        }
      }
      frame "2ndPrint" {
        n122 = Unbundle(w339) -> ("Dist. b/w cells line (mm)"=w346:dbl[], "Pitch (mm)"=w345:dbl[], "Num. of Drops"=w344:dbl, "Dist. b/w wells (mm)"=w343:dbl[], "Num. of wells"=w342:dbl, "Num. of columns"=w341:dbl, "Dist. b/w Columns (mm)"=w340:dbl[])
        n123 = Wait (ms)(milliseconds to wait=u32 500) -> ()  [unwired: 1 out]
        n124 = call "Line_distance.vi"("Num. of Drops in"=w344, "Pitch in"=w345, "Dist. b/w Lines in"=w343) -> ("Array"=w349:dbl[])  [unwired: 8 in]
        n125 = call "POS?.vi"("All axes?"=TRUE, "Axis identifier?"=FALSE) -> ("Position"=w350:dbl[])  [unwired: 3 in, 14 out]
        n126 = for {
          N: w341 -> [_]
          tunnel: w350 -> [w359]
          tunnel: w344 -> [w362]
          tunnel: w345 -> [w361]
          tunnel: w349 -> [w360]
          tunnel: w347 -> [w358]
          tunnel: w342 -> [w357]
          tunnel: w340 -> [w356]
          i -> [w375]
          n127 = Not Equal To 0?(x=w375) -> (x != 0?=w370:bool)
          n128 = for {
            N: w357 -> [_]
            tunnel: w362 -> [w382]
            tunnel: w361 -> [w386]
            tunnel: w360 -> [w385]
            tunnel: w358 -> [w384]
            i -> [w387]
            n129 = flat-sequence {
              tunnel: w387 -> [w390]
              tunnel: w385 -> [w389]
              tunnel: [w388] -> w383
              tunnel: w383 -> [w403]
              tunnel: w382 -> [w416]
              tunnel: w386 -> [w415]
              tunnel: w384 -> [w414]
              tunnel: w382 -> [w413]
              frame #0 {
                n130 = Not Equal To 0?(x=w390) -> (x != 0?=w388:bool)
                n131 = case shown="False" w388 {
                  tunnel: w389 -> [w398 w400]
                  tunnel: [w397 w400] -> w392
                  frame False {
                    n132 = Multiply(x=w398, y=0.0) -> (x*y=w397:dbl[])
                  }
                  frame True {
                  }
                }
                n133 = call "MVR.vi"("Axes to move"=string[] ["1"], "Position values"=w392, "No.of digits"=i16 4) -> ()  [unwired: 2 in, 15 out]
                n134 = call "General wait for movement to stop.vi"("All axes?"=TRUE, "Additional wait time, ms"=u32 100, "Polling cycle \ntime, ms"=u32 1 ("Polling cycle \ntime, ms")) -> ()  [unwired: 5 in, 12 out]
              }
              frame #1 {
                n135 = case shown="False" w403 {
                  tunnel: dbl[] [10.0] ("Position values") -> [w410 w412]
                  tunnel: [w409 w412] -> w401
                  frame False {
                    n136 = Multiply(x=w410, y=0.0) -> (x*y=w409:dbl[])
                  }
                  frame True {
                  }
                }
                n137 = call "MVR.vi"("Axes to move"=string[] ["3"], "Position values"=w401, "No.of digits"=i16 4) -> ()  [unwired: 2 in, 15 out]
                n138 = call "General wait for movement to stop.vi"("All axes?"=TRUE, "Additional wait time, ms"=u32 100, "Polling cycle \ntime, ms"=u32 1 ("Polling cycle \ntime, ms")) -> ()  [unwired: 5 in, 12 out]
              }
              frame #2 {
                n139 = for {
                  N: w416 -> [_]
                  tunnel: w415 -> [w420]
                  tunnel: w414 -> [w419]
                  tunnel: w413 -> [w417]
                  i -> [w422]
                  n140 = Decrement(x=w417) -> (x-1=w418:dbl)
                  n141 = flat-sequence {
                    tunnel: w419 -> [w423]
                    tunnel: w421 -> [w426]
                    tunnel: w420 -> [w425]
                    frame #0 {
                      n142 = invoke class="bfx_piezo_r13" method="Shoot"(reference=w423) -> ()  [unwired: 2 in, 3 out]
                      n143 = Wait (ms)(milliseconds to wait=u32 200) -> ()  [unwired: 1 out]
                    }
                    frame #1 {
                      n144 = case shown="False" w426 {
                        tunnel: w425 -> [w427 _]
                        frame False {
                          n145 = call "MVR.vi"("Axes to move"=string[] ["1"], "Position values"=w427, "No.of digits"=i16 4) -> ()  [unwired: 2 in, 15 out]
                          n146 = call "General wait for movement to stop.vi"("All axes?"=TRUE, "Additional wait time, ms"=u32 100, "Polling cycle \ntime, ms"=u32 1 ("Polling cycle \ntime, ms")) -> ()  [unwired: 5 in, 12 out]
                        }
                        frame True {
                          n147 = call "MVR.vi"("Axes to move"=string[] ["3"], "Position values"=dbl[] [-10.0], "No.of digits"=i16 4) -> ()  [unwired: 2 in, 15 out]
                          n148 = call "General wait for movement to stop.vi"("All axes?"=TRUE, "Additional wait time, ms"=u32 100, "Polling cycle \ntime, ms"=u32 1 ("Polling cycle \ntime, ms")) -> ()  [unwired: 5 in, 12 out]
                        }
                      }
                    }
                  }
                  n149 = Equal?(x=w418, y=w422) -> (x = y?=w421:bool)
                }
              }
            }
          }
          n150 = case shown="False" w370 {
            tunnel: w356 -> [w377 w381]
            tunnel: [w376 w380] -> w369
            frame False {
              n151 = Multiply(x=w377, y=0.0) -> (x*y=w376:dbl[])
            }
            frame True {
              n152 = Multiply(x=w381, y=dbl[] [-1.0]) -> (x*y=w380:dbl[])
            }
          }
          n153 = call "MVR.vi"("Axes to move"=string[] ["2"], "Position values"=w369, "No.of digits"=i16 4) -> ()  [unwired: 2 in, 15 out]
          n154 = call "General wait for movement to stop.vi"("All axes?"=TRUE, "Additional wait time, ms"=u32 100, "Polling cycle \ntime, ms"=u32 1 ("Polling cycle \ntime, ms")) -> ()  [unwired: 5 in, 12 out]
          n155 = call "MOV.vi"("Axes to move"=string[] ["1"], "Position values"=w359, "No.of digits"=i16 4) -> ()  [unwired: 2 in, 15 out]
          n156 = call "General wait for movement to stop.vi"("All axes?"=TRUE, "Additional wait time, ms"=u32 100, "Polling cycle \ntime, ms"=u32 1 ("Polling cycle \ntime, ms")) -> ()  [unwired: 5 in, 12 out]
        }
      }
      frame "AbsoluteCentering" {
        w440 = string[] ["1", "2", "3"] ("Axes to move")
        n157 = call "MOV.vi"("Axes to move"=w440, "Position values"="Position values (mm)", "No.of digits"=i16 4, "error in"=w446) -> ("error out"=w449:errorcluster)  [unwired: 1 in, 14 out]
        n158 = call "ONT?.vi"("Axes to query"=w440, "error in"=w449) -> ("error out"=w445:errorcluster)  [unwired: 3 in, 14 out]
        n159 = call "General wait for movement to stop.vi"("Axes to wait for"=w440, "Additional wait time, ms"=u32 100, "Polling cycle \ntime, ms"=u32 1 ("Polling cycle \ntime, ms")) -> ()  [unwired: 5 in, 12 out]
      }
      frame "RelativeCentering" {
        w459 = string[] ["3"] ("Axes to move")
        w467 = string[] ["2"] ("Axes to move")
        w468 = string[] ["1"] ("Axes to move")
        n160 = case shown="False" "Y-" {
          tunnel: "Y-Step Size (mm)" -> [w502 w505]
          tunnel: [w501 w504] -> w471
          frame False {
            n161 = Multiply(x=dbl[] [0.0], y=w502) -> (x*y=w501:dbl[])
          }
          frame True {
            n162 = Multiply(x=dbl[] [-1.0], y=w505) -> (x*y=w504:dbl[])
          }
        }
        n163 = case shown="False" "Y+" {
          tunnel: "Y-Step Size (mm)" -> [w496 w499]
          tunnel: [w495 w498] -> w470
          frame False {
            n164 = Multiply(x=dbl[] [0.0], y=w496) -> (x*y=w495:dbl[])
          }
          frame True {
            n165 = Multiply(x=dbl[] [1.0], y=w499) -> (x*y=w498:dbl[])
          }
        }
        n166 = case shown="True" "Z+" {
          tunnel: "Z-Step Size (mm)" -> [w490 w493]
          tunnel: [w489 w492] -> w462
          frame False {
            n167 = Multiply(x=dbl[] [0.0], y=w490) -> (x*y=w489:dbl[])
          }
          frame True {
            n168 = Multiply(x=dbl[] [-1.0], y=w493) -> (x*y=w492:dbl[])
          }
        }
        n169 = case shown="False" "X-" {
          tunnel: "X-Step Size (mm)" -> [w513 w517]
          tunnel: [w514 w516] -> w473
          frame False {
            n170 = Multiply(x=dbl[] [0.0], y=w513) -> (x*y=w514:dbl[])
          }
          frame True {
            n171 = Multiply(x=dbl[] [-1.0], y=w517) -> (x*y=w516:dbl[])
          }
        }
        n172 = case shown="False" "Z-" {
          tunnel: "Z-Step Size (mm)" -> [w484 w487]
          tunnel: [w483 w486] -> w461
          frame False {
            n173 = Multiply(x=dbl[] [0.0], y=w484) -> (x*y=w483:dbl[])
          }
          frame True {
            n174 = Multiply(x=dbl[] [1.0], y=w487) -> (x*y=w486:dbl[])
          }
        }
        n175 = case shown="False" "X+" {
          tunnel: "X-Step Size (mm)" -> [w508 w511]
          tunnel: [w507 w510] -> w472
          frame False {
            n176 = Multiply(x=dbl[] [0.0], y=w508) -> (x*y=w507:dbl[])
          }
          frame True {
            n177 = Multiply(x=dbl[] [1.0], y=w511) -> (x*y=w510:dbl[])
          }
        }
        n178 = call "MVR.vi"("Axes to move"=w467, "Position values"=w471) -> ()  [unwired: 3 in, 15 out]
        n179 = call "MVR.vi"("Axes to move"=w467, "Position values"=w470) -> ()  [unwired: 3 in, 15 out]
        n180 = call "MVR.vi"("Axes to move"=w468, "Position values"=w472) -> ()  [unwired: 3 in, 15 out]
        n181 = call "MVR.vi"("Axes to move"=w459, "Position values"=w462) -> ()  [unwired: 3 in, 15 out]
        n182 = call "MVR.vi"("Axes to move"=w459, "Position values"=w461) -> ()  [unwired: 3 in, 15 out]
        n183 = call "MVR.vi"("Axes to move"=w468, "Position values"=w473) -> ()  [unwired: 3 in, 15 out]
        n184 = call "General wait for movement to stop.vi"("Axes to wait for"=w468, "Polling cycle \ntime, ms"=u32 1 ("Polling cycle \ntime, ms")) -> ()  [unwired: 6 in, 12 out]
        n185 = call "General wait for movement to stop.vi"("Axes to wait for"=w467, "Polling cycle \ntime, ms"=u32 1 ("Polling cycle \ntime, ms")) -> ()  [unwired: 6 in, 12 out]
        n186 = call "General wait for movement to stop.vi"("Axes to wait for"=w467, "Polling cycle \ntime, ms"=u32 1 ("Polling cycle \ntime, ms")) -> ()  [unwired: 6 in, 12 out]
        n187 = call "General wait for movement to stop.vi"("Axes to wait for"=w459, "Polling cycle \ntime, ms"=u32 1 ("Polling cycle \ntime, ms")) -> ()  [unwired: 6 in, 12 out]
        n188 = call "General wait for movement to stop.vi"("Axes to wait for"=w459, "Polling cycle \ntime, ms"=u32 1 ("Polling cycle \ntime, ms")) -> ()  [unwired: 6 in, 12 out]
        n189 = call "General wait for movement to stop.vi"("Axes to wait for"=w468, "Polling cycle \ntime, ms"=u32 1 ("Polling cycle \ntime, ms")) -> ()  [unwired: 6 in, 12 out]
      }
    }
  }
  "error out" <- w2
